vi "Read Position.vi"(8 "error in (no error)":errorcluster, 11 "Amphipod in":refnum<class "Amphipod.lvclass">) -> (0 "error out":errorcluster, 2 "Position":cluster{"Row":i8, "Column":i8}, 3 "Amphipod out":refnum<class "Amphipod.lvclass">)   [LabVIEW 2019, in "23.lvlib" / "Amphipod.lvclass"]
uses:
  Amphipod.lvclass
  Amphipod.lvclass/Amphipod.ctl
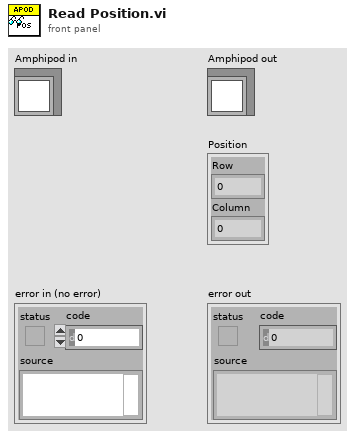
[diagram p1: front panel]
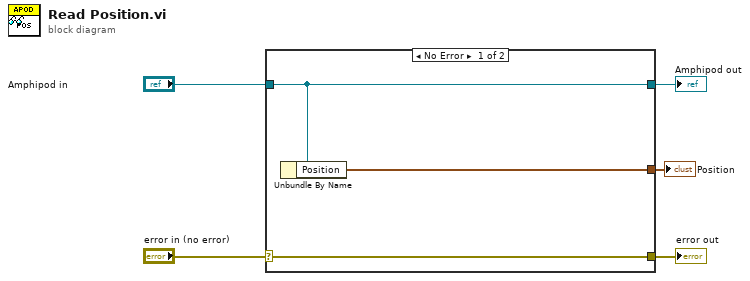
[diagram p0: block diagram]
diagram:
  n1 = case shown="No Error" "error in (no error)" {
    selector: "error in (no error)" -> [w8 w9]
    tunnel: [w8 w9] -> w4
    tunnel: [w7 w10] -> w2
    tunnel: "Amphipod in" -> [w7 w10]
    tunnel: [w6 _] -> w1
    frame No Error {
      n2 = Unbundle By Name(w7) -> ("Position"=w6:cluster{"Row":i8, "Column":i8})
    }
    frame Error {
    }
  }
  "error out" <- w4
  "Amphipod out" <- w2
  "Position" <- w1
